vi "CMI ADS127L21 - Reset Timestamp.vi"(8 "error in (no error)":errorcluster, 11 "session in":T1) -> (0 "error out":errorcluster, 3 "session out":T1)   [LabVIEW 2020]
doc: "Resets runtime ADC timestamp to reduce loss of precission when its value is to high."
uses:
  CMI ADS127L21 - Session.ctl
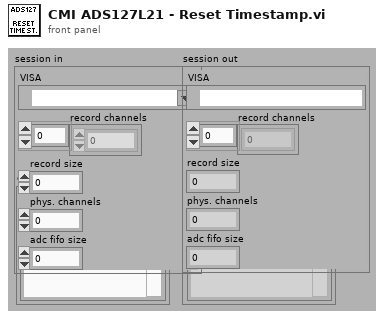
[diagram p1: front panel]
types:
  T1 = typedef "CMI ADS127L21 - Session.ctl" = cluster{"VISA":refnum<visa-resource-name>, "record channels":i32[], "record size":i32, "phys. channels":i32, "adc fifo size":i32}
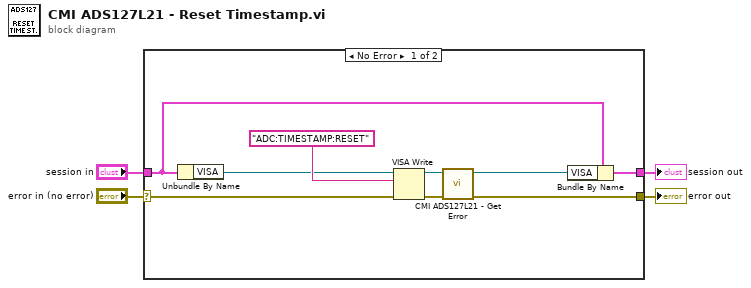
[diagram p0: block diagram]
diagram:
  n1 = case shown="No Error" "error in (no error)" {
    selector: "error in (no error)" -> [w9 w15]
    tunnel: "session in" -> [w5 w14]
    tunnel: [w6 w14] -> w3
    tunnel: [w10 w15] -> w2
    frame No Error {
      n2 = Unbundle By Name(w5) -> ("VISA"=w7:refnum<visa-resource-name>)
      n3 = VISA Write(VISA resource name=w7, write buffer="ADC:TIMESTAMP:RESET" ("format string"), error in (no error)=w9) -> (VISA resource name out=w12:refnum<visa-resource-name>, error out=w13:errorcluster)  [unwired: 1 out]
      n4 = call "CMI ADS127L21 - Get Error.vi"("error in (no error)"=w13, "VISA in"=w12) -> ("error out"=w10:errorcluster, "VISA out"=w11:refnum<visa-resource-name>)  [unwired: 8 in]
      n5 = Bundle By Name(cluster=w5, "VISA"=w11) -> (w6:T1)
    }
    frame Error {
    }
  }
  "error out" <- w2
  "session out" <- w3
